vi "E2_Control.vi"() -> ()   [LabVIEW 2019]
uses:
  <vilib>/Instr/_visa.llb/VISA Configure Serial Port (Instr).vi
  Instrument.Element2.lvclass
panel:
  out "Response":string
  out "read buffer":string
  in  "OpenLog":bool
  in  "UpdateTime":bool
  in  "ClearShutdown":bool
  in  "ClearWakeup":bool
  in  "Custom String":string
  in  "SendCustom":bool
  in  "ClearErrors":bool
  in  "Set Shutdown":bool
  in  "Shutdown Time":timestamp
  in  "Wakeup Time":timestamp
  in  "Set Wakeup":bool
  in  "Stop":bool
  in  "Start":bool
  in  "Write Buffer":string
  out "Laser":string
  out "Pump":string
  in  "Disconnect":bool
  in  "VISA Resource Name":refnum<visa-resource-name>
  in  "Resource Name":refnum<visa-resource-name>="Element2"
  in  "Status":bool
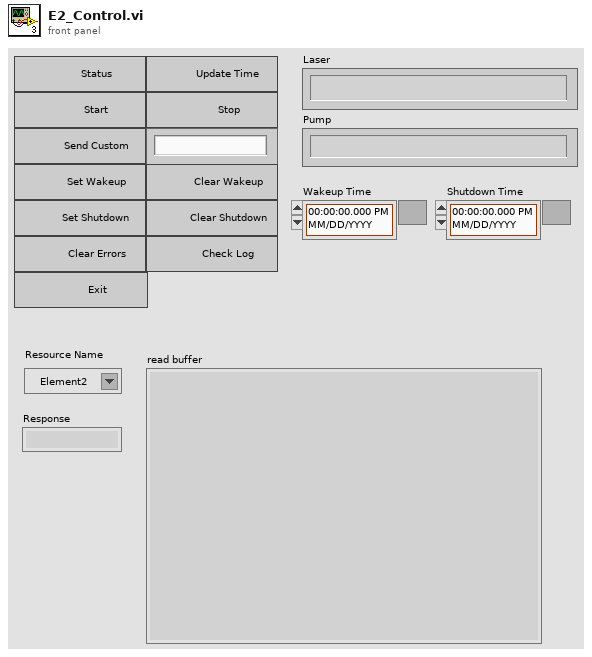
[diagram p1: front panel]
types:
  T1 = enum32{"Invalid", "Standard", "Closed", "Hidden", "Minimized", "Maximized"}
  T2 = enum32{"invalid app kind", "Development System", "Run Time System", "Student Edition", "Embedded LabVIEW", "Evaluation", "Custom"}
  T3 = enum16{"open", "replace", "create", "open or create", "replace or create", "replace or create with confirmation"}
  T4 = cluster{"Core":cluster{"Current VI Reference":refnum<vi>, "Close Panel on Exit?":bool}, "Your Boolean data":bool, "Your string data":string, "VISA Resource Name":refnum<visa-resource-name>, "Write Buffer":string, "Laser Status":string, "Pump Status":string}
  T5 = cluster{"Current VI Reference":refnum<vi>, "Close Panel on Exit?":bool}
  T6 = cluster{"Firmware":string, "[1]":string, "Serial No.":string, "[3]":string, "Laser Hrs.":string, "Year (YYYY)":string, "Month (MM)":string, "Date (DD)":string, "Hours (hh)":string, "Minutes (mm)":string, "Seconds (ss)":string, "[11]":string, "[12]":string, "Laser Status":string, "[14]":string, "Startup/Shutdown Status":string, "[16]":string, "[17]":string, "[18]":string, "[19]":string, "[20]":string, "[21]":string, "[22]":string, "[23]":string, "[24]":string, "[25]":string, "[26]":string, "Pico Speed":string, "Pico #":string, "[29]":string, "[30]":string, "[31]":string, "[32]":string, "[33]":string, "[34]":string, "[35]":string, "[36]":string, "[37]":string, "[38]":string, "[39]":string, "[40]":string, "[41]":string, "[42]":string, "[43]":string, "[44]":string, "[45]":string, "[46]":string, "[47]":string, "[48]":string, "[49]":string, "[50]":string, "[51]":string, "[52]":string, "[53]":string, "[54]":string, "[55]":string, "[56]":string, "[57]":string, "[58]":string, "[59]":string, "[60]":string, "[61]":string, "[62]":string, "[63]":string, "[64]":string, "[65]":string, "[66]":string, "[67]":string, "[68]":string, "[69]":string, "[70]":string, "[71]":string, "[72]":string, "[73]":string, "[74]":string, "Pump Laser 1":string, "Pump Laser 2":string, "Pump Laser 3":string, "Pump Laser 4":string, "Pump Laser 5":string, "[80]":string, "[81]":string, "[82]":string, "[83]":string, "[84]":string, "Diode Current Set":string, "Diode Current Actual":string, "[87]":string, "Pump Power":string, "[89]":string, "[90]":string, "[91]":string, "Temp: Pump Chassis":string, "Temp: Pump Diodes":string, "Temp: Pump Tower":string, "Temp: Pump PCB":string, "SHG Point":string, "[97]":string, "[98]":string, "[99]":string, "[100]":string, "[101]":string, "[102]":string, "Spectrometer: Int. time":string, "[104]":string, "[105]":string, "[106]":string, "Starter: Duration":string, "Starter: Voltage":string, "Starter: PWM Mode":string, "Starter: Duty Cycle":string, "PowSensCtrlLoop: Kp":string, "PowSensCtrlLoop: Ki":string, "Cycle Time":string, "Max Pump Current":string, "Loop Status":string, "CrysPos: Move Interval":string, "CrysPos: Pico Steps":string, "CrysPos: Step Direction":string, "CrysPos: Max Moves":string, "CrysPos: Last Move":string, "CrysPos: Moves Done":string, "Temp: Control Unit":string, "Temp: Laser Head Pos 1":string, "Temp: Laser Head Pos 2":string, "[125]":string, "[126]":string, "[127]":string, "[128]":string, "[129]":string, "[130]":string, "[131]":string, "[132]":string, "[133]":string, "[134]":string, "[135]":string, "[136]":string, "[137]":string, "[138]":string, "[139]":string, "[140]":string, "[141]":string, "Wedge Control Counter":string, "[143]":string}
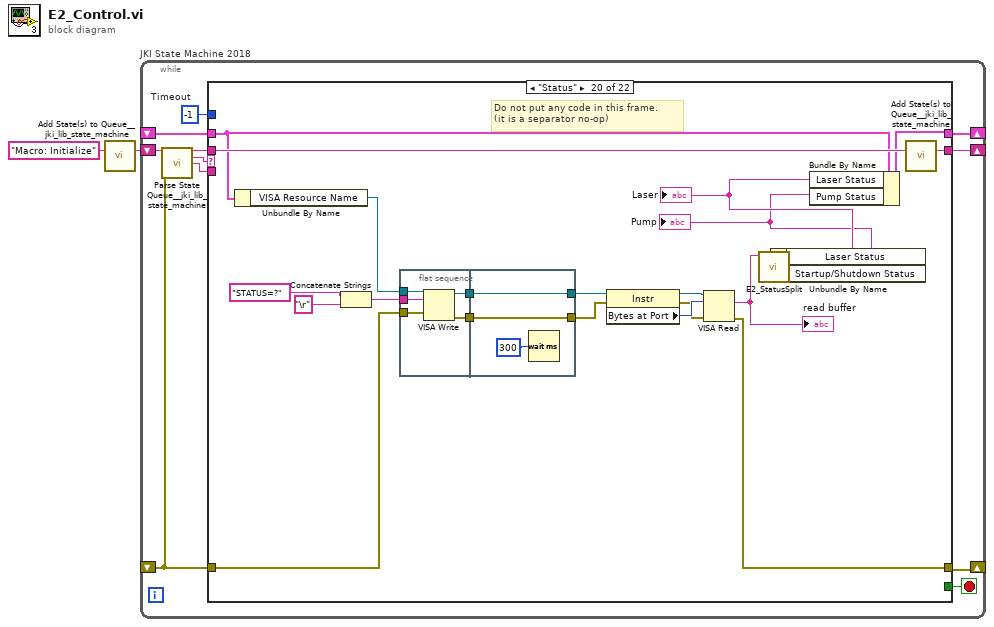
[diagram p0: block diagram]
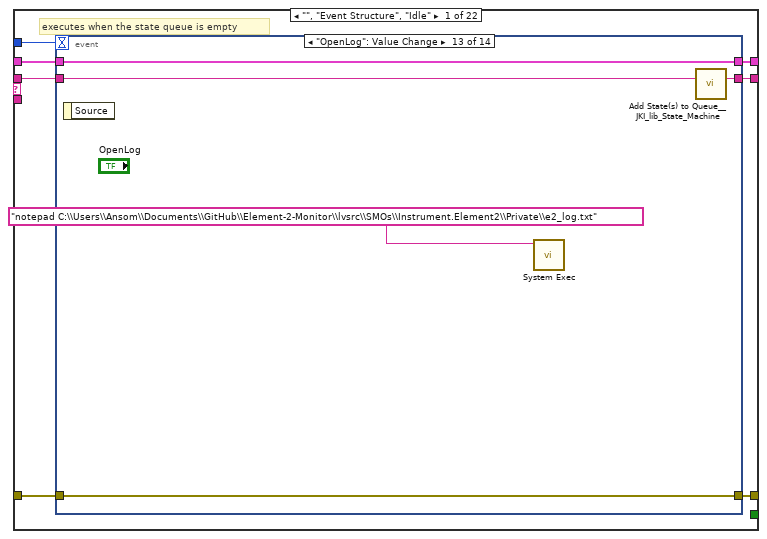
[diagram p2: hidden frame]
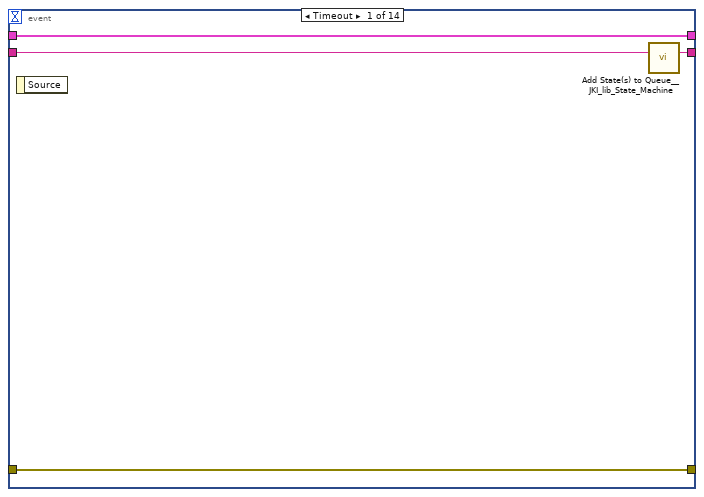
[diagram p3: hidden frame]
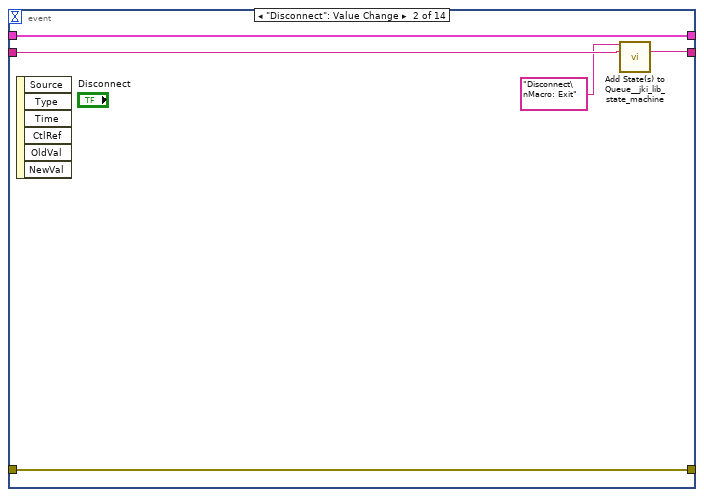
[diagram p4: hidden frame]
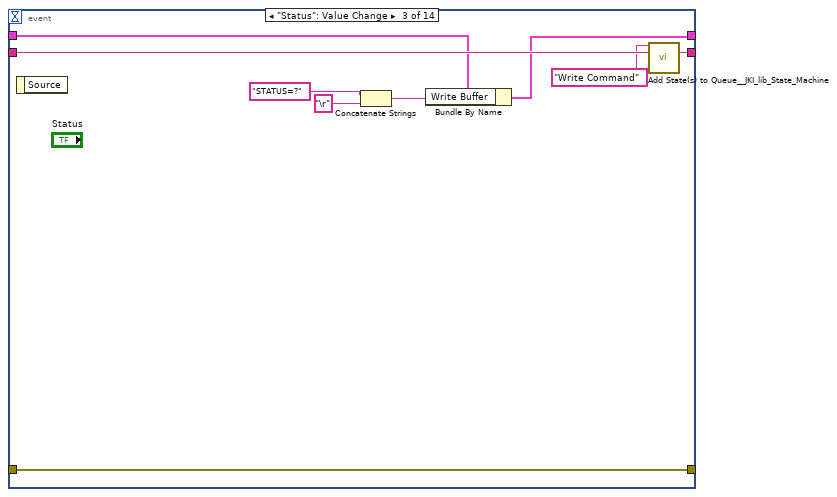
[diagram p5: hidden frame]
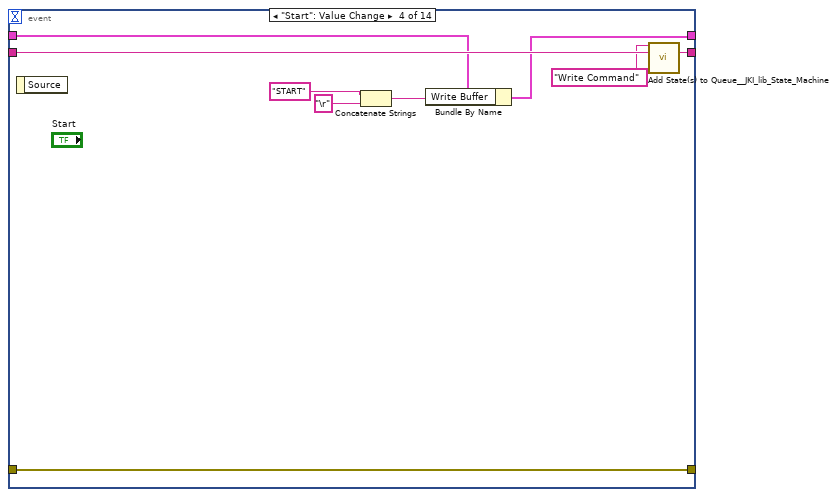
[diagram p6: hidden frame]
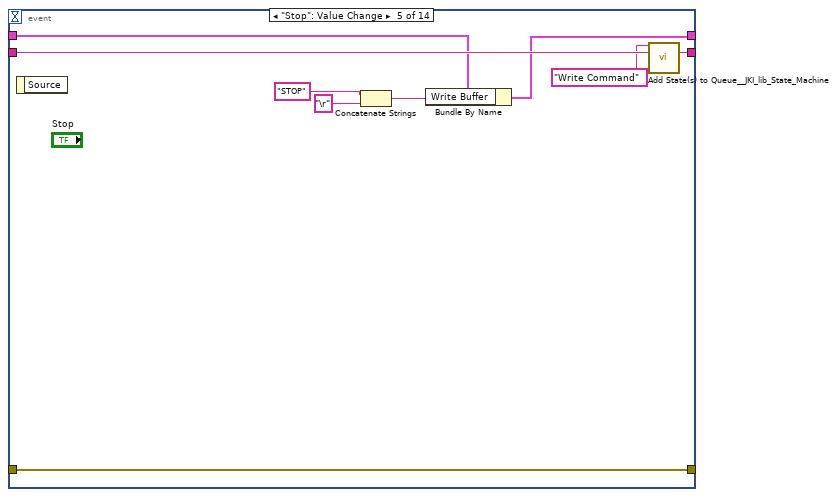
[diagram p7: hidden frame]
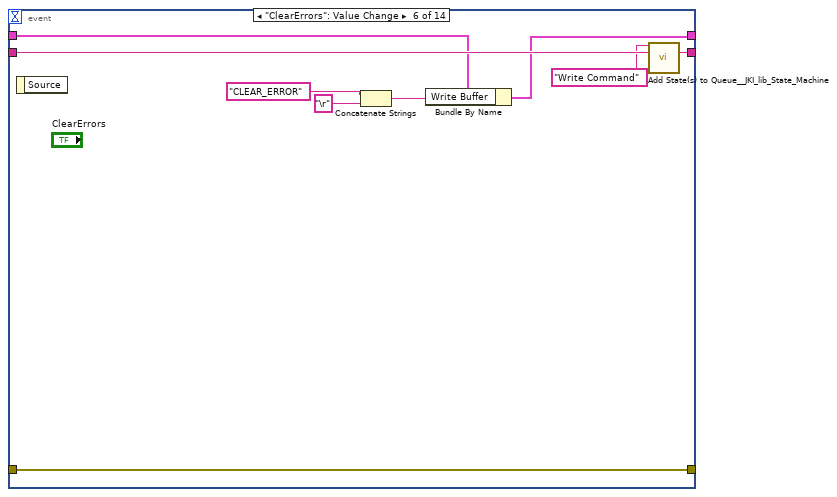
[diagram p8: hidden frame]
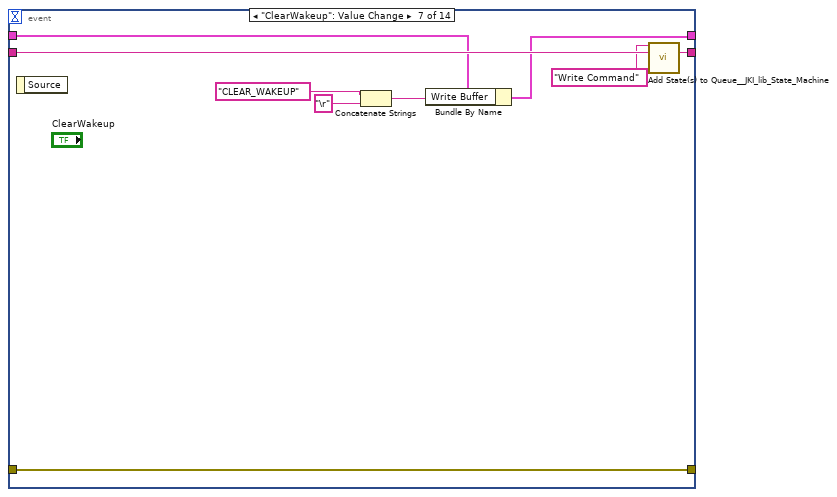
[diagram p9: hidden frame]
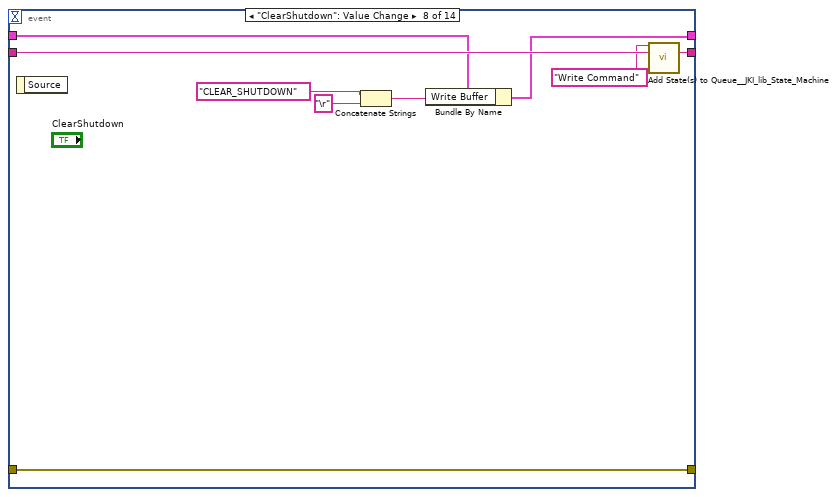
[diagram p10: hidden frame]
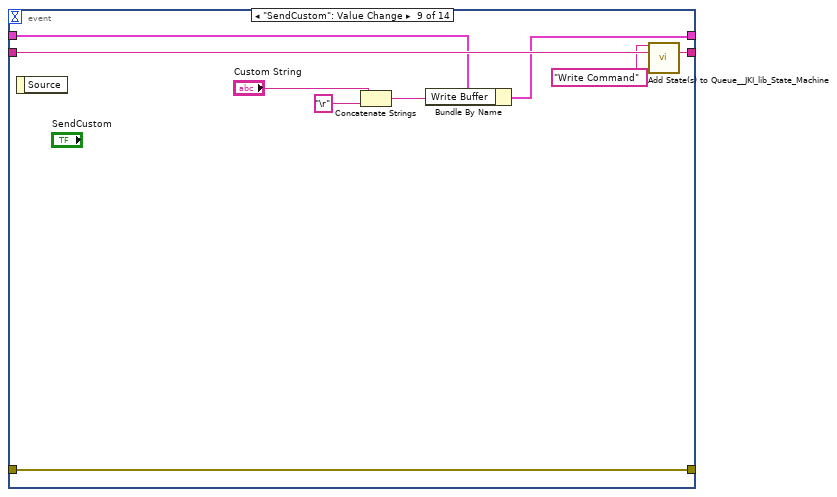
[diagram p11: hidden frame]
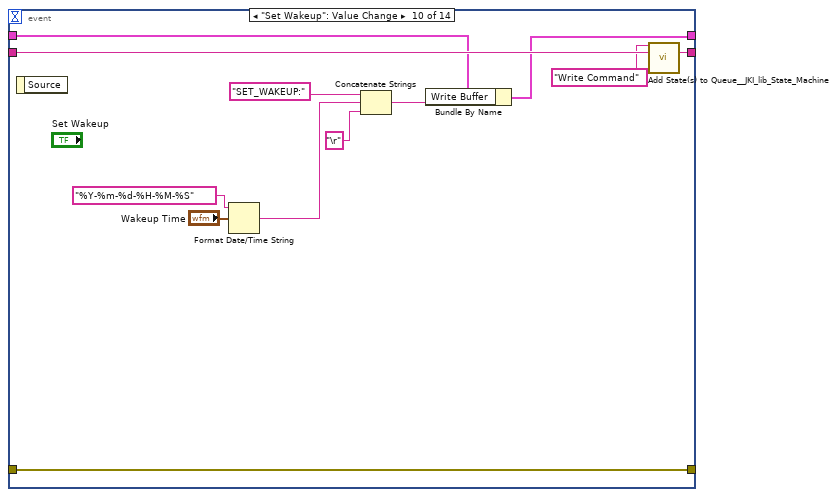
[diagram p12: hidden frame]
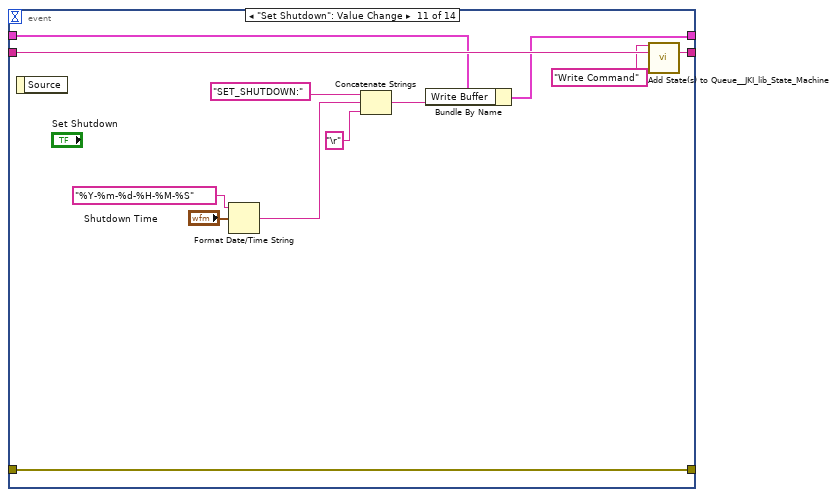
[diagram p13: hidden frame]
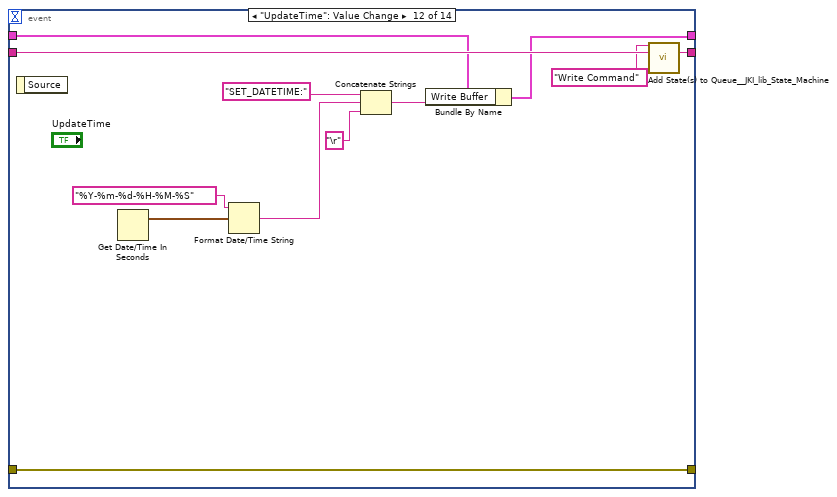
[diagram p14: hidden frame]
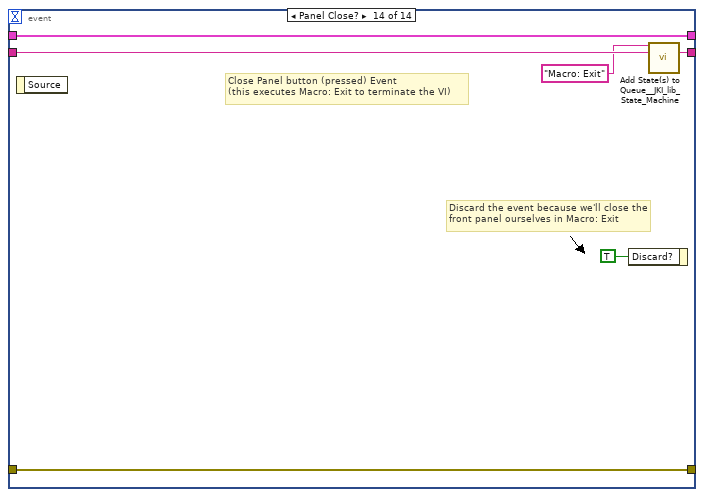
[diagram p15: hidden frame]
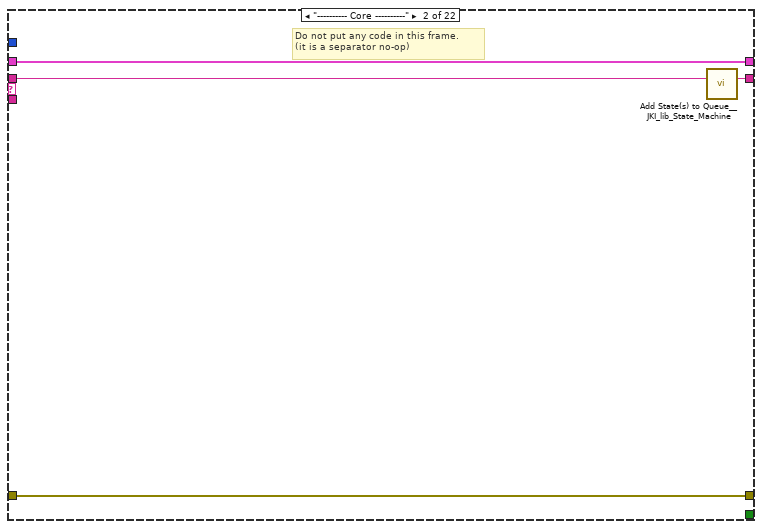
[diagram p16: hidden frame]
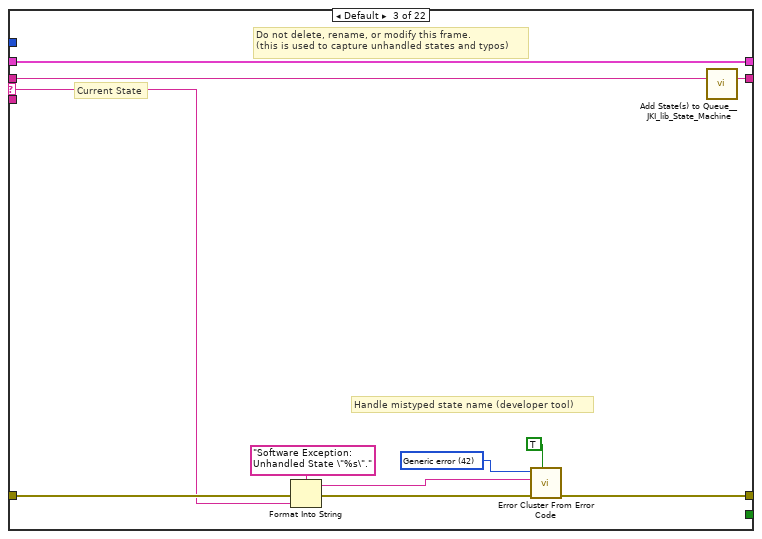
[diagram p17: hidden frame]
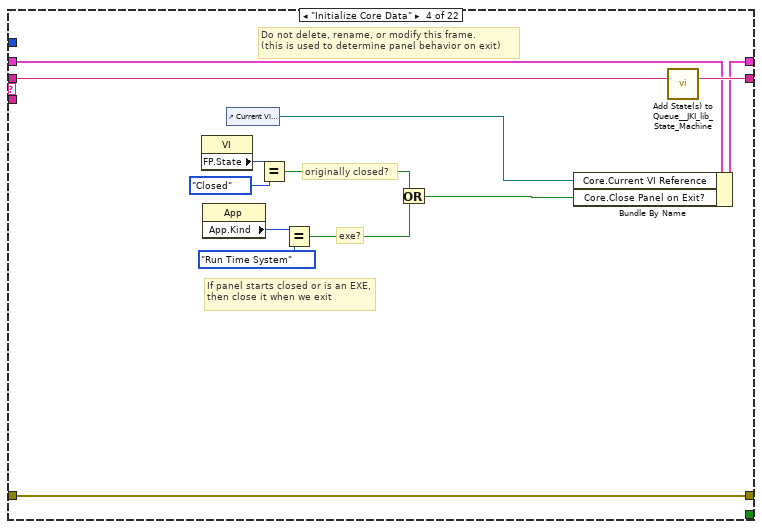
[diagram p18: hidden frame]
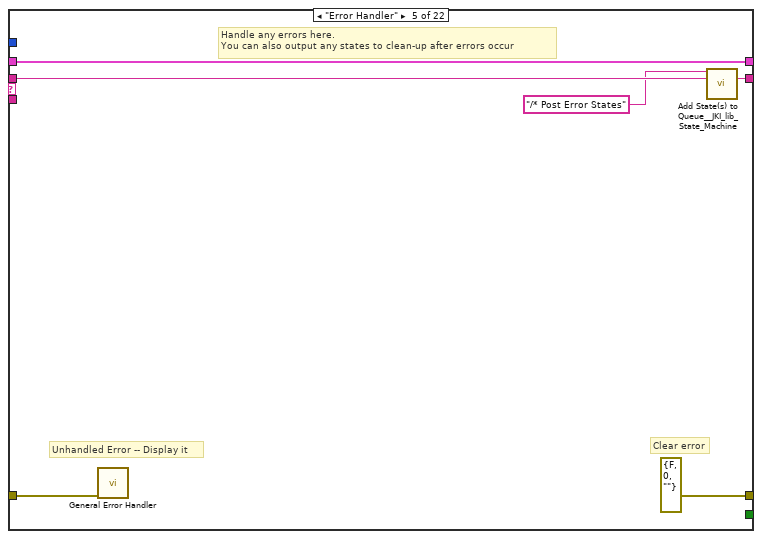
[diagram p19: hidden frame]
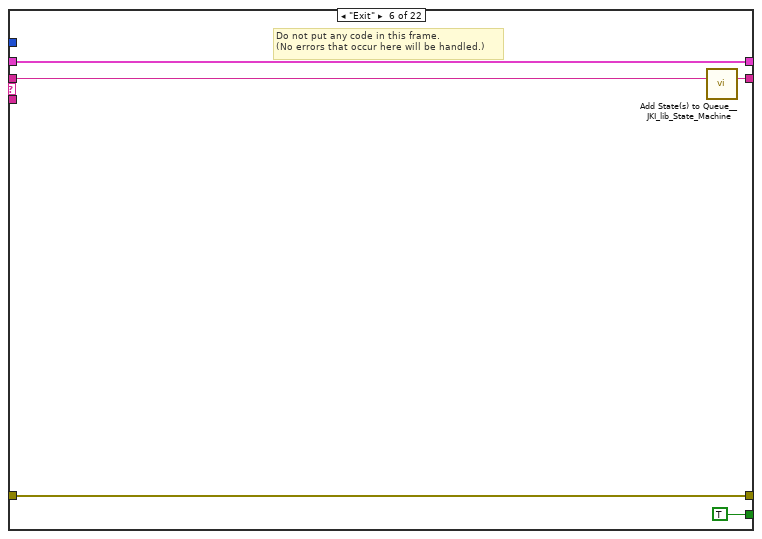
[diagram p20: hidden frame]
diagram:
  n1 = call <vilib>:"Add State(s) to Queue__jki_lib_state_machine.vi"("State(s) in (\"\")"="Macro: Initialize") -> ("States Out"=w2:string)  [unwired: 14 in]
  n2 = while "JKI State Machine 2018" {
    shift-right: [w6] -> _
    shift-left: _ -> [w5]
    shift-right: [w9] -> _
    shift-left: _ -> [w3]
    shift-right: [w8] -> _
    shift-left: w2 -> [w10]
    stop <- w7 stop-if-true
    w4 = -1  # Timeout
    n3 = call <vilib>:"Parse State Queue__jki_lib_state_machine.vi"("State Queue"=w10, "Error In (no error)"=w3) -> ("Remaining States"=w12:string, "Current State"=w13:string, "Arguments"=w11:string)  [unwired: 11 in]
    n4 = case shown="\"Status\"" w13 {
      selector: w13 -> [_ _ w144 _ _ _ _ _ _ _ _ _ _ _ _ _ _ _ _ _ _ _]
      tunnel: w12 -> [w20 w143 w148 w167 w173 w178 w182 w193 w199 w203 w207 w213 w224 w293 w298 w308 w312 w327 w335 w356 w380 w409]
      tunnel: w11 -> [_ _ _ _ _ _ _ _ _ _ _ w208 w218 _ _ _ _ _ _ _ _ _]
      tunnel: w5 -> [w18 w140 w146 w160 w170 w176 w179 _ w194 w200 w205 w211 w220 w290 w295 w305 w309 w319 w329 w341 w378 w405]
      tunnel: [w17 w141 w150 w164 errorcluster {"status"=FALSE, "code"=0, "source"=""} ("error out") w175 w180 w190 w195 w201 w204 w209 w221 w291 w296 w306 w310 w315 w331 w345 w371 w395] -> w9
      tunnel: w3 -> [w16 w141 w149 w164 w169 w175 w180 w190 w196 w201 w204 w210 w222 w291 w296 w306 w310 w316 w330 w350 w376 w396]
      tunnel: [w19 w142 w147 w166 w172 w177 w181 w192 w198 w202 w206 w212 w223 w292 w297 w307 w311 w326 w334 w355 w379 w408] -> w8
      tunnel: [_ _ _ _ _ TRUE _ _ _ _ _ _ _ _ _ _ _ _ _ _ _ _] -> w7
      tunnel: [w15 w140 w146 w165 w170 w176 w179 w191 w194 w200 w205 w211 w220 w290 w295 w305 w309 w318 w329 w340 w378 w405] -> w6
      tunnel: w4 -> [w14 _ _ _ _ _ _ _ _ _ _ _ _ _ _ _ _ _ _ _ _ _]
      frame "", "Event Structure", "Idle" {
        # "executes when the state queue is empty"
        n5 = event shown="[12] \"OpenLog\": Value Change" {
          selector: _ -> [_ _ _ _ _ _ _ _ _ _ _ _ _ _]
          dyn-events: _ -> [_ _ _ _ _ _ _ _ _ _ _ _ _ _]
          timeout: w14 -> [_ _ _ _ _ _ _ _ _ _ _ _ _ _]
          tunnel: w20 -> [w24 w27 w38 w47 w56 w65 w74 w83 w92 w104 w116 w128 w133 w139]
          tunnel: [w23 w28 w37 w46 w55 w64 w73 w82 w91 w103 w115 w127 w132 w138] -> w19
          tunnel: w18 -> [w21 w29 w34 w43 w52 w61 w70 w79 w88 w100 w112 w124 w130 w136]
          tunnel: [w22 w25 w36 w45 w54 w63 w72 w81 w90 w102 w114 w126 w131 w137] -> w17
          tunnel: w16 -> [w22 w25 w36 w45 w54 w63 w72 w81 w90 w102 w114 w126 w131 w137]
          tunnel: [w21 w29 w33 w42 w51 w60 w69 w78 w87 w99 w111 w123 w130 w136] -> w15
          event Timeout {
            n6 = event-data() -> ()  [unwired: 1 in, 1 out]
            n7 = call <vilib>:"Add State(s) to Queue__JKI_lib_State_Machine.vi"("State(s) in (\"\")"=w24) -> ("States Out"=w23:string)  [unwired: 14 in]
          }
          event "Disconnect": Value Change {
            n8 = event-data() -> ()  [unwired: 1 in, 6 out]
            n9 = call <vilib>:"Add State(s) to Queue__jki_lib_state_machine.vi"("State(s) in Front (\"\")"="Disconnect\nMacro: Exit" ("State(s) in Front (\"\")"), "State(s) in (\"\")"=w27) -> ("States Out"=w28:string)  [unwired: 13 in]
          }
          event "Status": Value Change {
            n10 = event-data() -> ()  [unwired: 1 in, 1 out]
            n11 = Concatenate Strings("STATUS=?" ("string"), "\r" ("string")) -> (w30:string)
            n12 = Bundle By Name(cluster=w34, "Write Buffer"=w30) -> (w33:T4)
            n13 = call <vilib>:"Add State(s) to Queue__JKI_lib_State_Machine.vi"("State(s) in Front (\"\")"="Write Command", "State(s) in (\"\")"=w38) -> ("States Out"=w37:string)  [unwired: 13 in]
          }
          event "Start": Value Change {
            n14 = event-data() -> ()  [unwired: 1 in, 1 out]
            n15 = Concatenate Strings("START" ("string"), "\r" ("string")) -> (w39:string)
            n16 = Bundle By Name(cluster=w43, "Write Buffer"=w39) -> (w42:T4)
            n17 = call <vilib>:"Add State(s) to Queue__JKI_lib_State_Machine.vi"("State(s) in Front (\"\")"="Write Command", "State(s) in (\"\")"=w47) -> ("States Out"=w46:string)  [unwired: 13 in]
          }
          event "Stop": Value Change {
            n18 = event-data() -> ()  [unwired: 1 in, 1 out]
            n19 = Concatenate Strings("STOP" ("string"), "\r" ("string")) -> (w48:string)
            n20 = Bundle By Name(cluster=w52, "Write Buffer"=w48) -> (w51:T4)
            n21 = call <vilib>:"Add State(s) to Queue__JKI_lib_State_Machine.vi"("State(s) in Front (\"\")"="Write Command", "State(s) in (\"\")"=w56) -> ("States Out"=w55:string)  [unwired: 13 in]
          }
          event "ClearErrors": Value Change {
            n22 = event-data() -> ()  [unwired: 1 in, 1 out]
            n23 = Concatenate Strings("CLEAR_ERROR" ("string"), "\r" ("string")) -> (w57:string)
            n24 = Bundle By Name(cluster=w61, "Write Buffer"=w57) -> (w60:T4)
            n25 = call <vilib>:"Add State(s) to Queue__JKI_lib_State_Machine.vi"("State(s) in Front (\"\")"="Write Command", "State(s) in (\"\")"=w65) -> ("States Out"=w64:string)  [unwired: 13 in]
          }
          event "ClearWakeup": Value Change {
            n26 = event-data() -> ()  [unwired: 1 in, 1 out]
            n27 = Concatenate Strings("CLEAR_WAKEUP" ("string"), "\r" ("string")) -> (w66:string)
            n28 = Bundle By Name(cluster=w70, "Write Buffer"=w66) -> (w69:T4)
            n29 = call <vilib>:"Add State(s) to Queue__JKI_lib_State_Machine.vi"("State(s) in Front (\"\")"="Write Command", "State(s) in (\"\")"=w74) -> ("States Out"=w73:string)  [unwired: 13 in]
          }
          event "ClearShutdown": Value Change {
            n30 = event-data() -> ()  [unwired: 1 in, 1 out]
            n31 = Concatenate Strings("CLEAR_SHUTDOWN" ("string"), "\r" ("string")) -> (w75:string)
            n32 = Bundle By Name(cluster=w79, "Write Buffer"=w75) -> (w78:T4)
            n33 = call <vilib>:"Add State(s) to Queue__JKI_lib_State_Machine.vi"("State(s) in Front (\"\")"="Write Command", "State(s) in (\"\")"=w83) -> ("States Out"=w82:string)  [unwired: 13 in]
          }
          event "SendCustom": Value Change {
            n34 = event-data() -> ()  [unwired: 1 in, 1 out]
            n35 = Concatenate Strings("Custom String", "\r" ("string")) -> (w85:string)
            n36 = Bundle By Name(cluster=w88, "Write Buffer"=w85) -> (w87:T4)
            n37 = call <vilib>:"Add State(s) to Queue__JKI_lib_State_Machine.vi"("State(s) in Front (\"\")"="Write Command", "State(s) in (\"\")"=w92) -> ("States Out"=w91:string)  [unwired: 13 in]
          }
          event "Set Wakeup": Value Change {
            n38 = event-data() -> ()  [unwired: 1 in, 1 out]
            n39 = Format Date/Time String(time format string (%c)="%Y-%m-%d-%H-%M-%S", seconds (now)="Wakeup Time") -> (date/time string=w93:string)  [unwired: 1 in]
            n40 = Concatenate Strings("SET_WAKEUP:" ("string"), w93, "\r" ("string")) -> (w97:string)
            n41 = Bundle By Name(cluster=w100, "Write Buffer"=w97) -> (w99:T4)
            n42 = call <vilib>:"Add State(s) to Queue__JKI_lib_State_Machine.vi"("State(s) in Front (\"\")"="Write Command", "State(s) in (\"\")"=w104) -> ("States Out"=w103:string)  [unwired: 13 in]
          }
          event "Set Shutdown": Value Change {
            n43 = event-data() -> ()  [unwired: 1 in, 1 out]
            n44 = Format Date/Time String(time format string (%c)="%Y-%m-%d-%H-%M-%S", seconds (now)="Shutdown Time") -> (date/time string=w105:string)  [unwired: 1 in]
            n45 = Concatenate Strings("SET_SHUTDOWN:" ("string"), w105, "\r" ("string")) -> (w109:string)
            n46 = Bundle By Name(cluster=w112, "Write Buffer"=w109) -> (w111:T4)
            n47 = call <vilib>:"Add State(s) to Queue__JKI_lib_State_Machine.vi"("State(s) in Front (\"\")"="Write Command", "State(s) in (\"\")"=w116) -> ("States Out"=w115:string)  [unwired: 13 in]
          }
          event "UpdateTime": Value Change {
            n48 = event-data() -> ()  [unwired: 1 in, 1 out]
            n49 = Get Date/Time In Seconds() -> (seconds since 1Jan1904=w117:timestamp)
            n50 = Format Date/Time String(time format string (%c)="%Y-%m-%d-%H-%M-%S", seconds (now)=w117) -> (date/time string=w118:string)  [unwired: 1 in]
            n51 = Concatenate Strings("SET_DATETIME:" ("string"), w118, "\r" ("string")) -> (w121:string)
            n52 = Bundle By Name(cluster=w124, "Write Buffer"=w121) -> (w123:T4)
            n53 = call <vilib>:"Add State(s) to Queue__JKI_lib_State_Machine.vi"("State(s) in Front (\"\")"="Write Command", "State(s) in (\"\")"=w128) -> ("States Out"=w127:string)  [unwired: 13 in]
          }
          event "OpenLog": Value Change {
            n54 = event-data() -> ()  [unwired: 1 in, 1 out]
            n55 = call <vilib>:"System Exec.vi"("command line"="notepad C:\\Users\\Ansom\\Documents\\GitHub\\Element-2-Monitor\\lvsrc\\SMOs\\Instrument.Element2\\Private\\e2_log.txt") -> ()  [unwired: 7 in, 4 out]
            n56 = call <vilib>:"Add State(s) to Queue__JKI_lib_State_Machine.vi"("State(s) in (\"\")"=w133) -> ("States Out"=w132:string)  [unwired: 14 in]
          }
          event Panel Close? {
            # "Discard the event because we'll close the front panel ourselves in Macro: Exit"
            # "Close Panel button (pressed) Event\n(this executes Macro: Exit to terminate the VI)"
            n57 = event-data() -> ()  [unwired: 1 in, 1 out]
            n58 = event-data("Discard?"=TRUE) -> ()  [unwired: 1 in, 1 out]
            n59 = call <vilib>:"Add State(s) to Queue__JKI_lib_State_Machine.vi"("State(s) in Front (\"\")"="Macro: Exit", "State(s) in (\"\")"=w139) -> ("States Out"=w138:string)  [unwired: 13 in]
          }
        }
      }
      frame "---------- Core ----------" {
        # "Do not put any code in this frame.\n(it is a separator no-op)"
        n60 = call <vilib>:"Add State(s) to Queue__JKI_lib_State_Machine.vi"("State(s) in (\"\")"=w143) -> ("States Out"=w142:string)  [unwired: 14 in]
      }
      frame Default {
        w153 = 42 items=["No error", "Argument error", "Memory is full", "Out of zone", "End of file", "File already open", "Generic file I/O error", "File not found", "File permission error", "Disk is full", "Duplicate path", "Too many files open", "System feature not enabled", "Resource file not found", "Cannot add resource", "Resource not found", "Image not found", "Image memory error", "Pen does not exist", "Config type invalid", "Config token not found", "Config parse error", "Config memory error", "Bad external code format", "Bad external code offset", "External code not present", "Null window", "Destroy window error", "Null menu", "Print aborted", "Bad print record", "Print driver error", "Windows error during printing", "Memory error during printing", "Print dialog error", "Generic print error", "Invalid device refnum", "Device not found", "Device parameter error", "Device unit error", "Cannot open device", "Device call aborted", "Generic error", "Cancelled by user", "Object ID too low", "Object ID too high", "Object not in heap", "Unknown heap", "Unknown object (invalid DefProc)", "Unknown object (DefProc not in table)", "Message out of range", "Invalid (null) method", "Unknown message", "Manager call not supported", "Bad address", "Network operation in progress", "Network operation timed out", "Connection is busy", "Network attribute not supported", "Network error", "Address in use", "System out of memory", "Connection aborted", "Connection refused", "Not connected", "Already connected", "Connection closed", "Initialization error (interapplication manager)", "Bad occurrence", "Wait on unbound occurrence handler", "Occurrence queue overflow", "Datalog type conflict", "Unused", "Unrecognized type (interapplication manager)", "Memory corrupt", "Failed to make temporary DLL", "Old CIN version", "Drag socket not found", "Failed to load drop-object", "Failed to register OLE object", "Failed to release OLE object", "Format specifier type mismatch", "Unknown format specifier", "Too few format specifiers", "Too many format specifiers", "Scan failed", "Newer CIN version", "Error converting to variant", "Runtime menu error", "Password tampered", "Variant attribute not found", "Incompatible variant data type", "Event data is not available", "Event Store is not present", "Occurrence is not found", "Event Queue is not created", "Event info is not available", "Refnum passed is NULL", "Error retrieving Class GUID", "Error retrieving CoClass GUID", "Error retrieving TypeLib GUID.", "Bad built application magic bytes.", "Specific driver is different from the specific driver associated with the Logical Name.", "There is no session opened to the class driver.", "Max Error", "MAX - Error with config objects", "MAX - Error loading configuration", "MAX - Group not supported"]
        # "Current State"
        # "Do not delete, rename, or modify this frame.\n(this is used to capture unhandled states and typos)"
        # "Handle mistyped state name (developer tool)"
        n61 = Format Into String(format string="Software Exception: Unhandled State \"%s\"." ("message"), error in=w149, w144) -> (resulting string=w152:string, error out=w151:errorcluster)  [unwired: 1 in]
        n62 = call <vilib>:"Error Cluster From Error Code.vi"("show call chain? (False)"=TRUE, "error in (no error)"=w151, "error message (\"\")"=w152, "error code (0)"=w153) -> ("error out"=w150:errorcluster)  [unwired: 5 in]
        n63 = call <vilib>:"Add State(s) to Queue__JKI_lib_State_Machine.vi"("State(s) in (\"\")"=w148) -> ("States Out"=w147:string)  [unwired: 14 in]
      }
      frame "Initialize Core Data" {
        # "Do not delete, rename, or modify this frame.\n(this is used to determine panel behavior on exit)"
        # "originally closed?"
        # "exe?"
        # "If panel starts closed or is an EXE, then close it when we exit"
        n64 = property class="VI"() -> ("FP.State"=w157:T1)  [unwired: 2 in, 2 out]
        n65 = property class="App"() -> ("App.Kind"=w163:T2)  [unwired: 2 in, 2 out]
        n66 = control-ref of="Current VI Reference"() -> (w158:refnum<vi>)
        n67 = Equal?(x=w157, y=T1."Closed" ("Front Panel Window:State")) -> (x = y?=w155:bool)
        n68 = Equal?(x=w163, y=T2."Run Time System" ("Application:Kind")) -> (x = y?=w161:bool)
        n69 = Or(x=w155, y=w161) -> (x .or. y?=w159:bool)
        n70 = Bundle By Name(cluster=w160, "Core.Current VI Reference"=w158, "Core.Close Panel on Exit?"=w159) -> (w165:T4)
        n71 = call <vilib>:"Add State(s) to Queue__JKI_lib_State_Machine.vi"("State(s) in (\"\")"=w167) -> ("States Out"=w166:string)  [unwired: 14 in]
      }
      frame "Error Handler" {
        # "Unhandled Error -- Display it"
        # "Handle any errors here.\nYou can also output any states to clean-up after errors occur"
        # "Clear error"
        n72 = call <vilib>:"General Error Handler.vi"("error in (no error)"=w169) -> ()  [unwired: 10 in, 5 out]
        n73 = call <vilib>:"Add State(s) to Queue__JKI_lib_State_Machine.vi"("State(s) in Front (\"\")"="/* Post Error States", "State(s) in (\"\")"=w173) -> ("States Out"=w172:string)  [unwired: 13 in]
      }
      frame "Exit" {
        # "Do not put any code in this frame.\n(No errors that occur here will be handled.)"
        n74 = call <vilib>:"Add State(s) to Queue__JKI_lib_State_Machine.vi"("State(s) in (\"\")"=w178) -> ("States Out"=w177:string)  [unwired: 14 in]
      }
      frame "---------- Data ----------" {
        # "Do not put any code in this frame.\n(It is a separator no-op. You can make a copy of this frame to create a new Data frame)"
        n75 = call <vilib>:"Add State(s) to Queue__JKI_lib_State_Machine.vi"("State(s) in (\"\")"=w182) -> ("States Out"=w181:string)  [unwired: 14 in]
      }
      frame "Data: Initialize" {
        w183 = ""  # Pump Status
        w184 = ""  # Laser Status
        w187 = T5 {"Current VI Reference"=refnum, "Close Panel on Exit?"=FALSE}  # Core
        w189 = TRUE  # Your Boolean data
        w188 = ""  # Your string data
        # "Initialize the shift-register data, here.\n(data names are defined by what you wire into the bundle function)"
        n76 = Bundle("Core"=w187, "Your Boolean data"=w189, "Your string data"=w188, "VISA Resource Name"="VISA Resource Name", "Write Buffer"="Write Buffer", "Laser Status"=w184, "Pump Status"=w183) -> (w191:T4)  [unwired: 1 in]
        n77 = call <vilib>:"Add State(s) to Queue__JKI_lib_State_Machine.vi"("State(s) in (\"\")"=w193) -> ("States Out"=w192:string)  [unwired: 14 in]
      }
      frame "Data: Cleanup" {
        # "Cleanup any data and references, here.\n(this is called automatically, by the Macro: Exit)"
        n78 = Unbundle By Name(w194) -> ("Core.Current VI Reference"=w197:refnum<vi>)
        n79 = Close Reference(reference=w197, error in (no error)=w196) -> (error out=w195:errorcluster)
        n80 = call <vilib>:"Add State(s) to Queue__JKI_lib_State_Machine.vi"("State(s) in (\"\")"=w199) -> ("States Out"=w198:string)  [unwired: 14 in]
      }
      frame "---------- UI ----------" {
        # "Do not put any code in this frame.\n(It is a separator no-op. You can make a copy of this frame to create a new UI frame)"
        n81 = call <vilib>:"Add State(s) to Queue__JKI_lib_State_Machine.vi"("State(s) in (\"\")"=w203) -> ("States Out"=w202:string)  [unwired: 14 in]
      }
      frame "UI: Initialize" {
        # "Initialize the User Interface, here.\n(this is called automatically, by the Macro: Init)"
        n82 = call <vilib>:"Add State(s) to Queue__JKI_lib_State_Machine.vi"("State(s) in (\"\")"=w207) -> ("States Out"=w206:string)  [unwired: 14 in]
      }
      frame "UI: Cursor Set" {
        # "Argument"
        # "Set and Unset Cursor Busy.\n(Usage: \"UI: Cursor Set >> Busy|Idle\")"
        n83 = case shown="\"Idle\", Default" w208 {
          tunnel: w210 -> [w215 w217]
          tunnel: [w214 w216] -> w209
          frame "Idle", Default {
            n84 = call <vilib>:"Unset Busy.vi"("error in (no error)"=w215) -> ("error out"=w214:errorcluster)  [unwired: 10 in]
          }
          frame "Busy" {
            n85 = call <vilib>:"Set Busy.vi"("error in (no error)"=w217) -> ("error out"=w216:errorcluster)  [unwired: 9 in, 1 out]
          }
        }
        n86 = call <vilib>:"Add State(s) to Queue__JKI_lib_State_Machine.vi"("State(s) in (\"\")"=w213) -> ("States Out"=w212:string)  [unwired: 14 in]
      }
      frame "UI: Front Panel State" {
        # "Argument"
        # "Set Front Panel Open or Closed\n(Usage: \"UI: Front Panel State >> Open|Close\")"
        n87 = Unbundle By Name(w220) -> ("Core.Current VI Reference"=w219:refnum<vi>)
        n88 = case shown="\"Open\", \"Standard\", Default" w218 {
          tunnel: w222 -> [w230 w245 w256 w269 w282]
          tunnel: [w232 w246 w258 w271 w284] -> w221
          tunnel: w219 -> [w231 w243 w257 w270 w283]
          frame "Open", "Standard", Default {
            w225 = T1."Standard" ("State")
            n89 = property class="VI"(reference=w231, error in=w230) -> (reference out=w228:refnum<vi>, error out=w229:errorcluster, "FP.State"=w227:T1)
            n90 = Not Equal?(x=w227, y=w225) -> (x != y?=w226:bool)
            n91 = case shown="False" w226 {
              tunnel: [w236 w238] -> w232
              tunnel: w229 -> [w235 w238]
              tunnel: w228 -> [w234 _]
              tunnel: w225 -> [w233 _]
              frame True {
                n92 = invoke class="VI" method="FP.Open"(reference=w234, error in=w235, "Activate"=TRUE, "State"=w233) -> (error out=w236:errorcluster)  [unwired: 1 in, 4 out]
              }
              frame False {
              }
            }
          }
          frame "Close", "Closed" {
            n93 = property class="VI"(reference=w243, error in=w245) -> (reference out=w242:refnum<vi>, error out=w244:errorcluster, "FP.State"=w240:T1)
            n94 = Not Equal?(x=w240, y=T1."Closed" ("Front Panel Window:State")) -> (x != y?=w239:bool)
            n95 = case shown="True" w239 {
              tunnel: [w247 w250] -> w246
              tunnel: w244 -> [w247 w249]
              tunnel: w242 -> [_ w248]
              frame False {
              }
              frame True {
                n96 = invoke class="VI" method="FP.Close"(reference=w248, error in=w249) -> (error out=w250:errorcluster)  [unwired: 1 in, 2 out]
              }
            }
          }
          frame "Hidden", "Hide" {
            w251 = T1."Hidden" ("State")
            n97 = property class="VI"(reference=w257, error in=w256) -> (reference out=w254:refnum<vi>, error out=w255:errorcluster, "FP.State"=w253:T1)
            n98 = Not Equal?(x=w253, y=w251) -> (x != y?=w252:bool)
            n99 = case shown="True" w252 {
              tunnel: [w262 w263] -> w258
              tunnel: w255 -> [w261 w263]
              tunnel: w254 -> [w260 _]
              tunnel: w251 -> [w259 _]
              frame True {
                n100 = invoke class="VI" method="FP.Open"(reference=w260, error in=w261, "State"=w259) -> (error out=w262:errorcluster)  [unwired: 2 in, 4 out]
              }
              frame False {
              }
            }
          }
          frame "Minimize", "Minimized" {
            w264 = T1."Minimized" ("State")
            n101 = property class="VI"(reference=w270, error in=w269) -> (reference out=w267:refnum<vi>, error out=w268:errorcluster, "FP.State"=w266:T1)
            n102 = Not Equal?(x=w266, y=w264) -> (x != y?=w265:bool)
            n103 = case shown="True" w265 {
              tunnel: [w275 w276] -> w271
              tunnel: w268 -> [w274 w276]
              tunnel: w267 -> [w273 _]
              tunnel: w264 -> [w272 _]
              frame True {
                n104 = invoke class="VI" method="FP.Open"(reference=w273, error in=w274, "State"=w272) -> (error out=w275:errorcluster)  [unwired: 2 in, 4 out]
              }
              frame False {
              }
            }
          }
          frame "Maximize", "Maximized" {
            w277 = T1."Maximized" ("State")
            n105 = property class="VI"(reference=w283, error in=w282) -> (reference out=w280:refnum<vi>, error out=w281:errorcluster, "FP.State"=w279:T1)
            n106 = Not Equal?(x=w279, y=w277) -> (x != y?=w278:bool)
            n107 = case shown="True" w278 {
              tunnel: [w288 w289] -> w284
              tunnel: w281 -> [w287 w289]
              tunnel: w280 -> [w286 _]
              tunnel: w277 -> [w285 _]
              frame True {
                n108 = invoke class="VI" method="FP.Open"(reference=w286, error in=w287, "State"=w285) -> (error out=w288:errorcluster)  [unwired: 2 in, 4 out]
              }
              frame False {
              }
            }
          }
        }
        n109 = call <vilib>:"Add State(s) to Queue__JKI_lib_State_Machine.vi"("State(s) in (\"\")"=w224) -> ("States Out"=w223:string)  [unwired: 14 in]
      }
      frame "---------- Macro ----------" {
        # "Do not put any code in this frame.\n(It is a separator no-op. You can make a copy of this frame to create a new Macro frame)"
        n110 = call <vilib>:"Add State(s) to Queue__JKI_lib_State_Machine.vi"("State(s) in (\"\")"=w293) -> ("States Out"=w292:string)  [unwired: 14 in]
      }
      frame "Macro: Initialize" {
        w294 = "Data: Initialize\nInitialize Core Data\nUI: Initialize\nUI: Front Panel State >> Open\nInitialize"  # Data: Initialize Initialize Core Data UI: Initialize UI: Front Panel State >> Open Initialize
        # "Initialization Macro\n(This is called once, when the VI starts)"
        n111 = call <vilib>:"Add State(s) to Queue__JKI_lib_State_Machine.vi"("State(s) in Front (\"\")"=w294, "State(s) in (\"\")"=w298) -> ("States Out"=w297:string)  [unwired: 13 in]
      }
      frame "Macro: Exit" {
        # "Exit Macro\n(This is called once, when the VI exits)"
        n112 = Unbundle By Name(w305) -> ("Core.Close Panel on Exit?"=w304:bool)
        n113 = Select(t="UI: Front Panel State >> Close", s=w304, f="") -> (s? t:f=w301:string)
        n114 = call <vilib>:"Add State(s) to Queue__JKI_lib_State_Machine.vi"("State(s) in (\"\")"=w301, "State(s) at Back (\"\")"="Data: Cleanup\nExit") -> ("States Out"=w299:string)  [unwired: 13 in]
        n115 = call <vilib>:"Add State(s) to Queue__JKI_lib_State_Machine.vi"("State(s) in Front (\"\")"=w299, "State(s) in (\"\")"=w308) -> ("States Out"=w307:string)  [unwired: 13 in]
      }
      frame "---------- Element2 ----------" {
        # "Template Separator\n(You can make a copy of, or modify, this frame)"
        n116 = call <vilib>:"Add State(s) to Queue__JKI_lib_State_Machine.vi"("State(s) in (\"\")"=w312) -> ("States Out"=w311:string)  [unwired: 14 in]
      }
      frame "Initialize" {
        w320 = u16 0 items=["None", "XON/XOFF", "RTS/CTS", "XON/XOFF & RTS/CTS", "DTR/DSR", "XON/XOFF & DTR/DSR"]  # flow control (0:none)
        w321 = u16 8  # data bits (8)
        w322 = u32 115200  # baud rate (9600)
        w323 = enum16{"None", "Odd", "Even", "Mark", "Space"}."None"  # parity (0:none)
        # "Do not put any code in this frame.\n(it is a separator no-op)"
        n117 = call-poly "VISA Configure Serial Port"("VISA resource name"="Resource Name", "timeout (10sec)"=u32 1000, "Enable Termination\nChar (T)"=TRUE ("Enable Termination\nChar (T)"), "baud rate (9600)"=w322, "data bits (8)"=w321, "parity (0:none)"=w323, "error in (no error)"=w316, "flow control (0:none)"=w320) -> ("VISA resource name out"=w317:refnum<visa-resource-name>, "error out"=w315:errorcluster)  [unwired: 6 out]
        n118 = Bundle By Name(cluster=w319, "VISA Resource Name"=w317) -> (w318:T4)
        n119 = call <vilib>:"Add State(s) to Queue__JKI_lib_State_Machine.vi"("State(s) in Front (\"\")"="Status" ("State(s) in Front (\"\")"), "State(s) in (\"\")"=w327) -> ("States Out"=w326:string)  [unwired: 13 in]
      }
      frame "Disconnect" {
        # "Do not put any code in this frame.\n(it is a separator no-op)"
        n120 = Unbundle By Name(w329) -> ("VISA Resource Name"=w328:refnum<visa-resource-name>)
        n121 = VISA Flush I/O Buffer(VISA resource name=w328, error in (no error)=w330) -> (VISA resource name out=w333:refnum<visa-resource-name>, error out=w332:errorcluster)  [unwired: 1 in]
        n122 = VISA Close(VISA resource name=w333, error in (no error)=w332) -> (error out=w331:errorcluster)
        n123 = call <vilib>:"Add State(s) to Queue__JKI_lib_State_Machine.vi"("State(s) in (\"\")"=w335) -> ("States Out"=w334:string)  [unwired: 14 in]
      }
      frame "Status" {
        # "Do not put any code in this frame.\n(it is a separator no-op)"
        n124 = Unbundle By Name(w341) -> ("VISA Resource Name"=w352:refnum<visa-resource-name>)
        n125 = Concatenate Strings("STATUS=?" ("string"), "\r" ("string")) -> (w351:string)
        n126 = flat-sequence {
          tunnel: w352 -> [w361]
          tunnel: w351 -> [w360]
          tunnel: w350 -> [w359]
          tunnel: [w358] -> w348
          tunnel: [w357] -> w346
          tunnel: [w363] -> w349
          tunnel: w348 -> [w363]
          tunnel: [w362] -> w347
          tunnel: w346 -> [w362]
          frame #0 {
            n127 = VISA Write(VISA resource name=w361, write buffer=w360, error in (no error)=w359) -> (VISA resource name out=w357:refnum<visa-resource-name>, error out=w358:errorcluster)  [unwired: 1 out]
          }
          frame #1 {
            n128 = Wait (ms)(milliseconds to wait=u32 300) -> ()  [unwired: 1 out]
          }
        }
        n129 = property class="Instr"(reference=w347, error in=w349) -> (reference out=w344:refnum<visa-resource-name>, error out=w342:errorcluster, "Bytes at Port"=w343:u32)
        n130 = VISA Read(VISA resource name=w344, byte count=w343, error in (no error)=w342) -> (read buffer=w339:string, error out=w345:errorcluster)  [unwired: 2 out]
        "read buffer" <- w339
        n131 = call "E2_StatusSplit.vi"("Input String"=w339) -> ("Output Cluster"=w338:T6)  [unwired: 10 in]
        n132 = Unbundle By Name(w338) -> ("Laser Status"=w337:string, "Startup/Shutdown Status"=w336:string)
        "Laser" <- w337
        "Pump" <- w336
        n133 = Bundle By Name(cluster=w341, "Laser Status"=w337, "Pump Status"=w336) -> (w340:T4)
        n134 = call <vilib>:"Add State(s) to Queue__jki_lib_state_machine.vi"("State(s) in (\"\")"=w356) -> ("States Out"=w355:string)  [unwired: 14 in]
      }
      frame "Write Command" {
        # "Do not put any code in this frame.\n(it is a separator no-op)"
        n135 = Unbundle By Name(w378) -> ("VISA Resource Name"=w377:refnum<visa-resource-name>, "Write Buffer"=w367:string)
        n136 = flat-sequence {
          tunnel: w377 -> [w385]
          tunnel: w376 -> [w384]
          tunnel: [w383] -> w374
          tunnel: [w382] -> w372
          tunnel: w367 -> [w381]
          tunnel: [w387] -> w375
          tunnel: w374 -> [w387]
          tunnel: [w386] -> w373
          tunnel: w372 -> [w386]
          frame #0 {
            n137 = VISA Write(VISA resource name=w385, write buffer=w381, error in (no error)=w384) -> (VISA resource name out=w382:refnum<visa-resource-name>, error out=w383:errorcluster)  [unwired: 1 out]
          }
          frame #1 {
            n138 = Wait (ms)(milliseconds to wait=u32 300) -> ()  [unwired: 1 out]
          }
        }
        n139 = property class="Instr"(reference=w373, error in=w375) -> (reference out=w370:refnum<visa-resource-name>, error out=w368:errorcluster, "Bytes at Port"=w369:u32)
        n140 = VISA Read(VISA resource name=w370, byte count=w369, error in (no error)=w368) -> (read buffer=→"Response":string, error out=w371:errorcluster)  [unwired: 2 out]
        n141 = call <vilib>:"Add State(s) to Queue__JKI_lib_State_Machine.vi"("State(s) in Front (\"\")"="Status\nCreate Log" ("State(s) in Front (\"\")"), "State(s) in (\"\")"=w380) -> ("States Out"=w379:string)  [unwired: 13 in]
      }
      frame "Create Log" {
        w390 = "\t" ("string")
        # "Set file mark to\nend of file"
        # "Do not put any code in this frame.\n(it is a separator no-op)"
        n142 = Unbundle By Name(w405) -> ("Laser Status"=w392:string, "Pump Status"=w391:string, "Write Buffer"=w389:string)
        n143 = Get Date/Time In Seconds() -> (seconds since 1Jan1904=w406:timestamp)
        n144 = Format Date/Time String(time format string (%c)="%Y-%m-%d-%H-%M-%S", seconds (now)=w406) -> (date/time string=w404:string)  [unwired: 1 in]
        n145 = Open/Create/Replace File(file path (use dialog)=path "C:/Users/Ansom/Documents/GitHub/Element-2-Monitor/lvsrc/SMOs/Instrument.Element2/Private/e2_log.txt" ("file (use dialog)"), error in=w396, operation (0:open)=T3."open or create") -> (refnum out=w400:refnum<file>, error out=w399:errorcluster)  [unwired: 3 in, 1 out]
        n146 = Concatenate Strings(w404, w390, w392, w391, w390, w389) -> (w394:string)
        n147 = Set File Position(offset (in bytes) (0)=i64 0, refnum=w400, from (0:start)=enum16{"start", "end", "current"}."end", error in=w399) -> (refnum out=w402:refnum<file>, error out=w403:errorcluster)
        n148 = Write to Text File(file (use dialog)=w402, text=w394, error in=w403) -> (error out=w395:errorcluster)  [unwired: 1 in, 2 out]
        n149 = call <vilib>:"Add State(s) to Queue__JKI_lib_State_Machine.vi"("State(s) in (\"\")"=w409) -> ("States Out"=w408:string)  [unwired: 14 in]
      }
    }
  }
